vi "Update RPC Template Accessor.vi"(8 "error in (no error)":errorcluster, 10 "Accessor Name":string, 11 "Server Library (Library Item) in":refnum<vi>) -> (0 "error out":errorcluster, 3 "Server Library (Library Item) out":refnum<vi>)   [LabVIEW 2019, in "gRPC Scripting Tools.lvlib"]
uses:
  gRPC Scripting Tools.lvlib
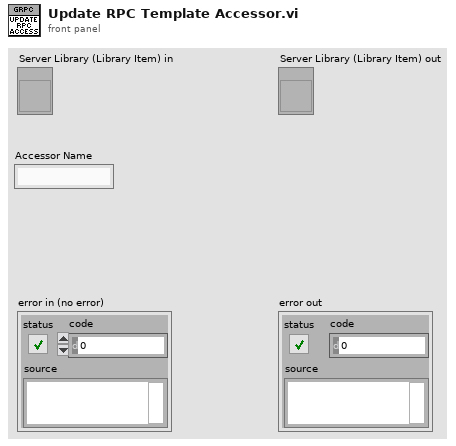
[diagram p1: front panel]
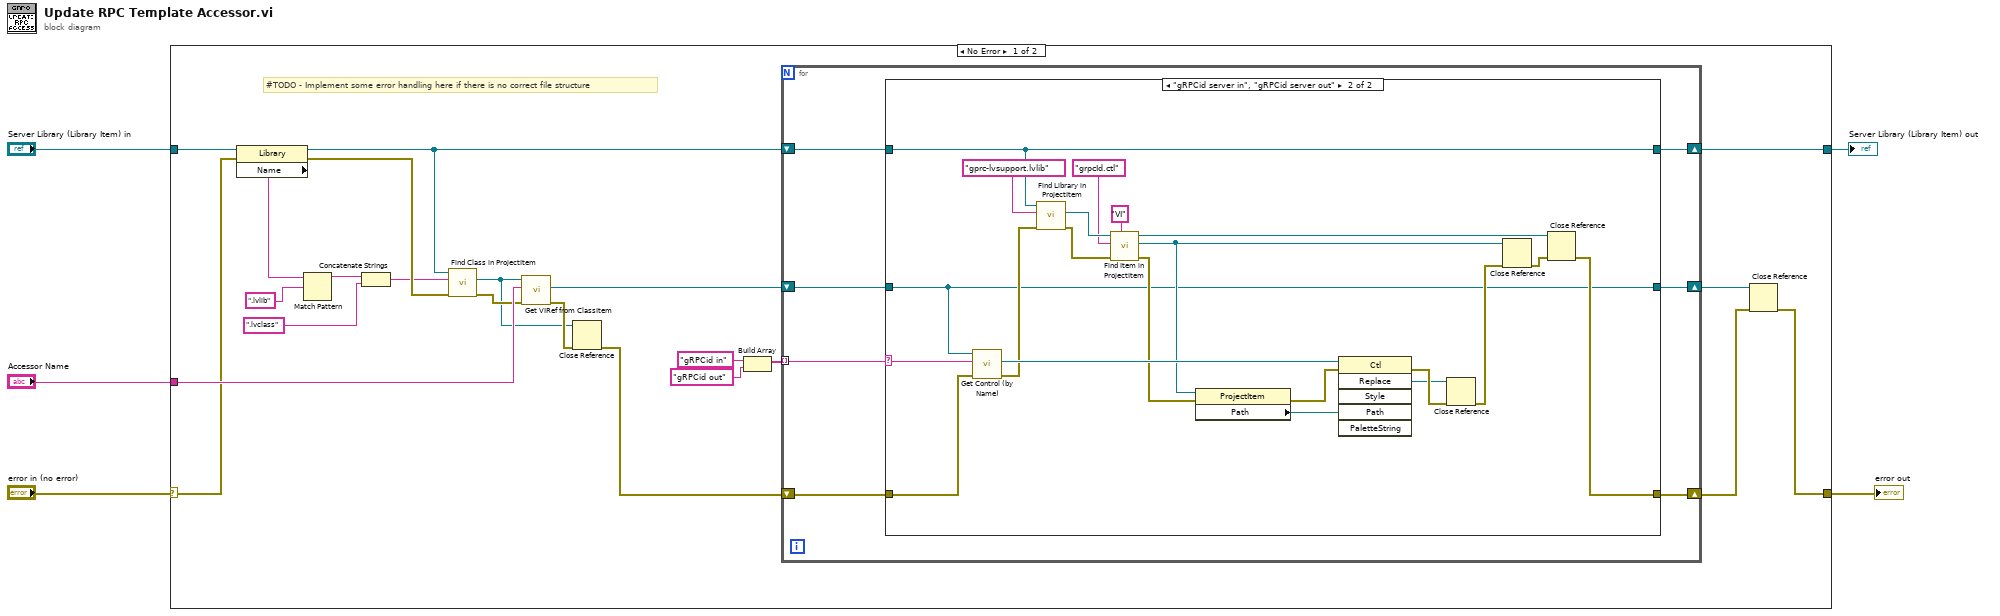
[diagram p0: block diagram]
diagram:
  n1 = case shown="No Error" "error in (no error)" {
    selector: "error in (no error)" -> [w10 w59]
    tunnel: [w27 w60] -> w5
    tunnel: "Server Library (Library Item) in" -> [w12 w60]
    tunnel: "Accessor Name" -> [w22 _]
    tunnel: [w19 w59] -> w2
    frame No Error {
      # "#TODO - Implement some error handling here if there is no correct file structure"
      n2 = property class="Library"(reference=w12, error in=w10) -> (reference out=w11:refnum<vi>, error out=w18:errorcluster, "Name"=w15:string)
      n3 = Match Pattern(string=w15, regular expression=".lvlib") -> (before substring=w16:string)  [unwired: 1 in, 3 out]
      n4 = Concatenate Strings(w16, ".lvclass" ("string")) -> (w17:string)
      n5 = call "Find Class in ProjectItem.vi"("error in (no error)"=w18, "Class Name"=w17, "ProjectItem in"=w11) -> ("error out"=w9:errorcluster, "LVClass out"=w7:refnum<vi>)  [unwired: 5 in, 2 out]
      n6 = call "Get VIRef from ClassItem.vi"("error in (no error)"=w9, "Item Name"=w22, "LVClassLibrary in"=w7) -> ("error out"=w8:errorcluster, "VIref out"=w23:refnum<vi>)  [unwired: 5 in, 2 out]
      n7 = Close Reference(reference=w7, error in (no error)=w8) -> (error out=w6:errorcluster)
      n8 = Build Array("gRPCid in" ("Item Name"), "gRPCid out" ("Item Name")) -> (w26:string[])
      n9 = for {
        tunnel: w26 -> [w34] mode=indexing
        shift-right: [w32] -> w27
        shift-left: w11 -> [w33]
        shift-right: [w29] -> w21
        shift-left: w6 -> [w30]
        shift-right: [w28] -> w20
        shift-left: w23 -> [w31]
        n10 = case shown="\"gRPCid server in\", \"gRPCid server out\"" w34 {
          selector: w34 -> [_ w41]
          tunnel: w33 -> [w37 w42]
          tunnel: [w37 w42] -> w32
          tunnel: w31 -> [w36 w38]
          tunnel: w30 -> [w35 w40]
          tunnel: [w35 w39] -> w29
          tunnel: [w36 w38] -> w28
          frame "False", Default {
          }
          frame "gRPCid server in", "gRPCid server out" {
            n11 = call "Get Control (by Name).vi"("error in (no error)"=w40, "Control Label"=w41, "Owner VI in"=w38) -> ("error out"=w52:errorcluster, "Control Refnum"=w54:refnum<vi>)  [unwired: 5 in, 2 out]
            n12 = call "Find Library in ProjectItem.vi"("error in (no error)"=w52, "Library Name"="gprc-lvsupport.lvlib", "ProjectItem in"=w42) -> ("error out"=w51:errorcluster, "Library out"=w57:refnum<vi>)  [unwired: 5 in, 2 out]
            n13 = call "Find Item in ProjectItem.vi"("Item Type"="VI", "error in (no error)"=w51, "Name"="grpcId.ctl", "ProjectItem in"=w57) -> ("error out"=w50:errorcluster, "Item Refnum out"=w45:refnum<vi>, "ProjectItem out"=w43:refnum<vi>)  [unwired: 4 in, 1 out]
            n14 = property class="ProjectItem"(reference=w45, error in=w50) -> (error out=w47:errorcluster, "Path"=w53:path)  [unwired: 1 out]
            n15 = invoke class="Ctl" method="Replace"(reference=w54, error in=w47, "Path"=w53) -> (error out=w49:errorcluster, "Replace"=w48:refnum<vi>)  [unwired: 3 in, 4 out]
            n16 = Close Reference(reference=w48, error in (no error)=w49) -> (error out=w46:errorcluster)
            n17 = Close Reference(reference=w45, error in (no error)=w46) -> (error out=w44:errorcluster)
            n18 = Close Reference(reference=w43, error in (no error)=w44) -> (error out=w39:errorcluster)
          }
        }
      }
      n19 = Close Reference(reference=w20, error in (no error)=w21) -> (error out=w19:errorcluster)
    }
    frame Error {
    }
  }
  "Server Library (Library Item) out" <- w5
  "error out" <- w2
